vi "rs3 get device.vi"(8 "error in":errorcluster, 10 "index":u32, 11 "context":u32) -> (0 "error out":errorcluster, 2 "device":u32, 3 "context":u64)   [LabVIEW 2017, in "libRealSense3.lvlib"]
doc: "Get the device handle needed for indexed device."
uses:
  <vilib>/addons/RealSense/libRealSense3.lvlib
  <vilib>/addons/RealSense/realsense-d.dll
panel:
  # "RS3 Get Device"
  # "(C) Intel Corp.,  AGJ"
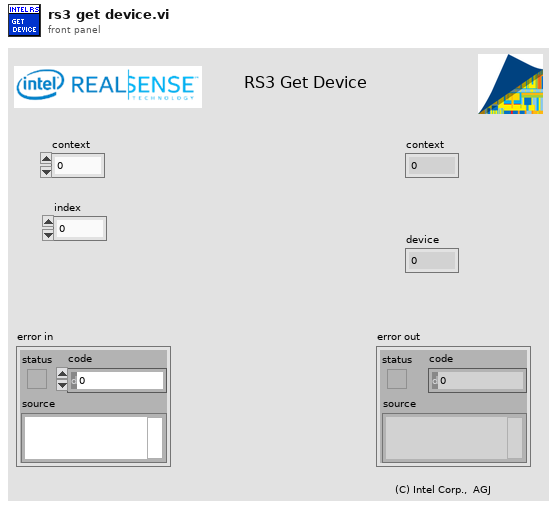
[diagram p1: front panel]
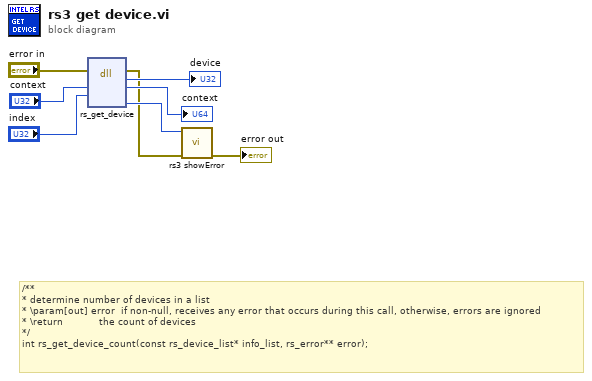
[diagram p0: block diagram]
diagram:
  # "/**\n* determine number of devices in a list\n* \\param[out] error  if non-null, receives any error that occurs during this call, otherwise, errors are ignored\n* \\return            the count of devices\n*/\nint rs_get_device_count(const rs_device_list* info_list, rs_error** error);"
  n1 = dll-call lib="C:/Program Files (x86)/National Instruments/LabVIEW 2017/vi.lib/addons/RealSense/realsense-d.dll" fn="rs_get_device"(error in="error in", "cxt"="context", "id"="index") -> (error out=w2:errorcluster, "device"=→"device":u32, "cxt"=→"context":u64, "error"=w3:u64)  [unwired: 4 in, 1 out]
  n2 = call <vilib>:"rs3 showError.vi"("error in (no error)"=w2, "error"=w3) -> ("error out"=→"error out":errorcluster)  [unwired: 5 in, 4 out]
